vi "Close Sessions_Controller_Screen.vi"(11 "Semiconductor Module Context":T1) -> (0 "error out":errorcluster)   [LabVIEW 2013]
uses:
  <vilib>/NI_TestStand_SemiconductorModule/NI_TestStand_Semiconductor_Module.lvlibp/PinMap/General/SemiconductorModuleContext.ctl
  <vilib>/NI_TestStand_SemiconductorModule/NI_TestStand_Semiconductor_Module.lvlibp
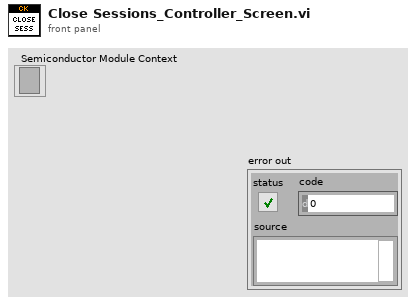
[diagram p1: front panel]
types:
  T1 = typedef "NI_TestStand_Semiconductor_Module.lvlibp/SemiconductorModuleContext.ctl" = refnum<k7>
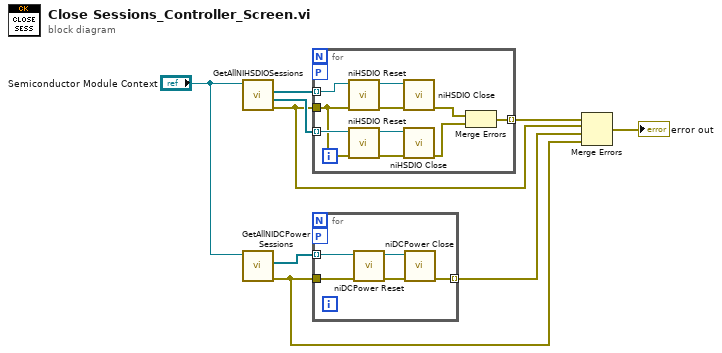
[diagram p0: block diagram]
diagram:
  n1 = call <vilib>:"GetAllNIHSDIOSessions.vi"("Semiconductor Module Context"="Semiconductor Module Context") -> ("error out"=w4:errorcluster, "Generation Sessions"=w8:refnum<k15>[], "Acquisition Sessions"=w9:refnum<k15>[])  [unwired: 7 in, 1 out]
  n2 = call <vilib>:"GetAllNIDCPowerSessions.vi"("Semiconductor Module Context"="Semiconductor Module Context") -> ("error out"=w2:errorcluster, "Instrument Sessions"=w7:refnum<k15>[])  [unwired: 8 in, 1 out]
  n3 = for {
    tunnel: w4 -> [w10]
    tunnel: w9 -> [w16] mode=indexing
    tunnel: w8 -> [w14] mode=indexing
    tunnel: [w11] -> w5 mode=indexing
    workers-P: _ -> [_]
    n4 = call <instrlib>:"niHSDIO Reset.vi"("error in (no error)"=w10, "instrument handle"=w16) -> ("error out"=w17:errorcluster, "instrument handle out"=w15:refnum<k15>)  [unwired: 8 in]
    n5 = call <instrlib>:"niHSDIO Reset.vi"("error in (no error)"=w10, "instrument handle"=w14) -> ("error out"=w19:errorcluster, "instrument handle out"=w18:refnum<k15>)  [unwired: 8 in]
    n6 = call <instrlib>:"niHSDIO Close.vi"("error in (no error)"=w17, "instrument handle"=w15) -> ("error out"=w13:errorcluster)  [unwired: 9 in]
    n7 = call <instrlib>:"niHSDIO Close.vi"("error in (no error)"=w19, "instrument handle"=w18) -> ("error out"=w12:errorcluster)  [unwired: 9 in]
    n8 = Merge Errors(w13, w12) -> (w11:errorcluster)
  }
  n9 = for {
    tunnel: w2 -> [w23]
    tunnel: w7 -> [w22] mode=indexing
    tunnel: [w24] -> w3 mode=indexing
    workers-P: _ -> [_]
    n10 = call <instrlib>:"niDCPower Reset.vi"("error in (no error)"=w23, "instrument handle"=w22) -> ("error out"=w20:errorcluster, "instrument handle out"=w21:refnum<k15>)  [unwired: 8 in]
    n11 = call <instrlib>:"niDCPower Close.vi"("error in (no error)"=w20, "instrument handle"=w21) -> ("error out"=w24:errorcluster)  [unwired: 9 in]
  }
  n12 = Merge Errors(w5, w4, w3, w2) -> (→"error out":errorcluster)
